vi "xunxian.vi"   [LabVIEW 2015]
uses:
  <vilib>/myRIO/Instrument Drivers/Onboard IO/DIO/typedefs/DIO Reference.ctl
  <vilib>/myRIO/Common/Instrument Driver Framework/Utilities/typedefs/myRIO Generic Hardware Reference.ctl
  <vilib>/myRIO/Common/Instrument Driver Framework/Utilities/typedefs/Hardware Version Enum.ctl
  <vilib>/myRIO/Common/Instrument Driver Framework/Utilities/typedefs/myRIO v1.0 Reference.ctl
  <vilib>/myRIO/Common/Instrument Driver Framework/Utilities/typedefs/Generic FPGA Reference.ctl
  <vilib>/myRIO/Common/Instrument Driver Framework/myRIO v1.0/DIO/typedefs/DIO Channels List.ctl
  <vilib>/myRIO/Common/Instrument Driver Framework/myRIO v1.0/DIO/typedefs/DIO Channels Enum.ctl
  <vilib>/userdefined/High Color/nirio_resource_hc.ctl
  <vilib>/myRIO/Instrument Drivers/Onboard IO/PWM/typedefs/PWM Reference.ctl
  <vilib>/myRIO/Common/Instrument Driver Framework/myRIO v1.0/PWM/typedefs/PWM Channels Enum.ctl
  <vilib>/myRIO/Instrument Drivers/Onboard IO/PWM/typedefs/PWM Configuration.ctl
  <vilib>/myRIO/Common/Instrument Driver Framework/Utilities/vis/Is FPGA Ref Available.vi
  <vilib>/myRIO/Common/Instrument Driver Framework/myRIO v1.0/DIO/vis/myRIO v1.1 Open DIO.vi
  <vilib>/myRIO/Instrument Drivers/Onboard IO/DIO/vis/Read.vi
  <vilib>/myRIO/Instrument Drivers/Onboard IO/DIO/vis/Write.vi
  <vilib>/myRIO/Common/Instrument Driver Framework/myRIO v1.0/PWM/vis/myRIO v1.1 Open PWM.vi
  <vilib>/myRIO/Instrument Drivers/Onboard IO/PWM/vis/Set Duty Cycle and Frequency.vi
  <vilib>/myRIO/Common/Instrument Driver Framework/Utilities/vis/Validate Channels.vi
  <vilib>/myRIO/Common/Instrument Driver Framework/myRIO v1.0/DIO/vis/myRIO v1.0 Reserve DIO.vi
  <vilib>/myRIO/Common/Instrument Driver Framework/myRIO v1.0/PWM/vis/myRIO v1.0 Reserve PWM.vi
  <vilib>/myRIO/Common/Instrument Driver Framework/myRIO v1.0/Resource Manager/vis/myRIO v1.0 Reserve Channel List.vi
  <vilib>/myRIO/Common/Instrument Driver Framework/myRIO v1.0/DIO/vis/myRIO v1.0 Build MUX Configuration DIO.vi
  <vilib>/myRIO/Common/Instrument Driver Framework/myRIO v1.0/PWM/vis/myRIO v1.0 Build MUX Configuration PWM.vi
  <vilib>/myRIO/Common/Instrument Driver Framework/myRIO v1.0/Resource Manager/vis/myRIO v1.0 Reserve Channel.vi
  <vilib>/myRIO/Common/Instrument Driver Framework/myRIO v1.0/Resource Manager/vis/myRIO v1.0 Unreserve Channel.vi
  <vilib>/myRIO/Common/Instrument Driver Framework/myRIO v1.0/Resource Manager/vis/myRIO v1.0 Create Configuration List.vi
  <vilib>/myRIO/Common/Instrument Driver Framework/myRIO v1.0/Resource Manager/vis/myRIO v1.0 Build Mutex Name.vi
  <vilib>/Utility/VariantDataType/GetNumericInfo.vi
  <vilib>/Utility/error.llb/Error Cluster From Error Code.vi
  <vilib>/myRIO/Common/Instrument Driver Framework/myRIO v1.0/myRIO v1.1 Open.vi
  <vilib>/myRIO/Common/Instrument Driver Framework/Utilities/vis/IO Manager.vi
  <vilib>/myRIO/Common/Instrument Driver Framework/Utilities/vis/Configuration Manager.vi
  <vilib>/myRIO/Common/Instrument Driver Framework/myRIO v1.0/Resource Manager/vis/myRIO v1.0 Configure IO.vi
  <vilib>/myRIO/Common/Instrument Driver Framework/myRIO v1.0/myRIO v1.0 Close.vi
  <vilib>/myRIO/Common/Instrument Driver Framework/myRIO v1.0/DIO/vis/myRIO v1.0 Write DIO.vi
  <vilib>/myRIO/Common/Instrument Driver Framework/myRIO v1.0/DIO/vis/myRIO v1.0 Read DIO.vi
  <vilib>/myRIO/Common/Instrument Driver Framework/myRIO v1.0/PWM/vis/myRIO v1.0 Write PWM.vi
  <vilib>/myRIO/Express VI/Onboard IO/DO/DO Express VI.xnode
  <vilib>/myRIO/Instrument Drivers/Onboard IO/DIO/vis/myRIO DIO Open.xnode
  <vilib>/myRIO/Express VI/Onboard IO/DI/DI Express VI.xnode
  <vilib>/myRIO/Express VI/Onboard IO/PWM/PWM Express VI.xnode
  <vilib>/myRIO/Instrument Drivers/Onboard IO/PWM/vis/myRIO PWM Open.xnode
  <vilib>/myRIO/Instrument Drivers/Onboard IO/PWM/PWM.lvlib
  <vilib>/myRIO/Instrument Drivers/Onboard IO/DIO/DIO.lvlib
types:
  T1 = typedef "DIO.lvlib/DIO Reference.ctl" = cluster{"myRIO Reference":T2, "DIO Channels List":T6}
  T2 = typedef "myRIO Generic Hardware Reference.ctl" = cluster{"myRIO Model":T3, "myRIO Hardware Reference":T4}
  T3 = typedef "Hardware Version Enum.ctl" = enum16{"Unknown", "myRIO-1900", "myRIO-1950", "roboRIO"}
  T4 = typedef "myRIO v1.0 Reference.ctl" = cluster{"Generic FPGA Reference":T5, "Allow multiple opens":bool}
  T5 = typedef "Generic FPGA Reference.ctl" = refnum<k20>
  T6 = typedef "DIO Channels List.ctl" = T7[]
  T7 = typedef "DIO Channels Enum.ctl" = enum16{"Not Connected", "C/DIO0", "C/DIO1", "C/DIO2", "C/DIO3", "C/DIO4", "C/DIO5", "C/DIO6", "C/DIO7", "A/DIO0", "A/DIO1", "A/DIO2", "A/DIO3", "A/DIO4", "A/DIO5", "A/DIO6", "A/DIO7", "A/DIO8", "A/DIO9", "A/DIO10", "A/DIO11", "A/DIO12", "A/DIO13", "A/DIO14", "A/DIO15", "B/DIO0", "B/DIO1", "B/DIO2", "B/DIO3", "B/DIO4", "B/DIO5", "B/DIO6", "B/DIO7", "B/DIO8", "B/DIO9", "B/DIO10", "B/DIO11", "B/DIO12", "B/DIO13", "B/DIO14", "B/DIO15", "LED0", "LED1", "LED2", "LED3", "Button0", "DIO/DIO0", "DIO/DIO1", "DIO/DIO2", "DIO/DIO3", "DIO/DIO4", "DIO/DIO5", "DIO/DIO6", "DIO/DIO7", "DIO/DIO8", "DIO/DIO9", "SPI/CS0", "SPI/CS1", "SPI/CS2", "SPI/CS3", "LED RADIO (Green)", "LED RADIO (Red)", "LED COMM (Green)", "LED COMM (Red)", "LED MODE (Green)", "LED MODE (Red)"}
  T8 = typedef "nirio_resource_hc.ctl" = tag
  T9 = typedef "PWM.lvlib/PWM Reference.ctl" = cluster{"myRIO Reference":T2, "PWM Channels Enum":T10, "PWM Configuration":T11}
  T10 = typedef "PWM Channels Enum.ctl" = enum16{"Not Connected", "C/PWM0", "C/PWM1", "A/PWM0", "A/PWM1", "A/PWM2", "B/PWM0", "B/PWM1", "B/PWM2", "PWM/PWM0", "PWM/PWM1", "PWM/PWM2", "PWM/PWM3", "PWM/PWM4", "PWM/PWM5", "PWM/PWM6", "PWM/PWM7", "PWM/PWM8", "PWM/PWM9"}
  T11 = typedef "PWM.lvlib/PWM Configuration.ctl" = cluster{"Frequency":dbl, "Duty Cycle":dbl}
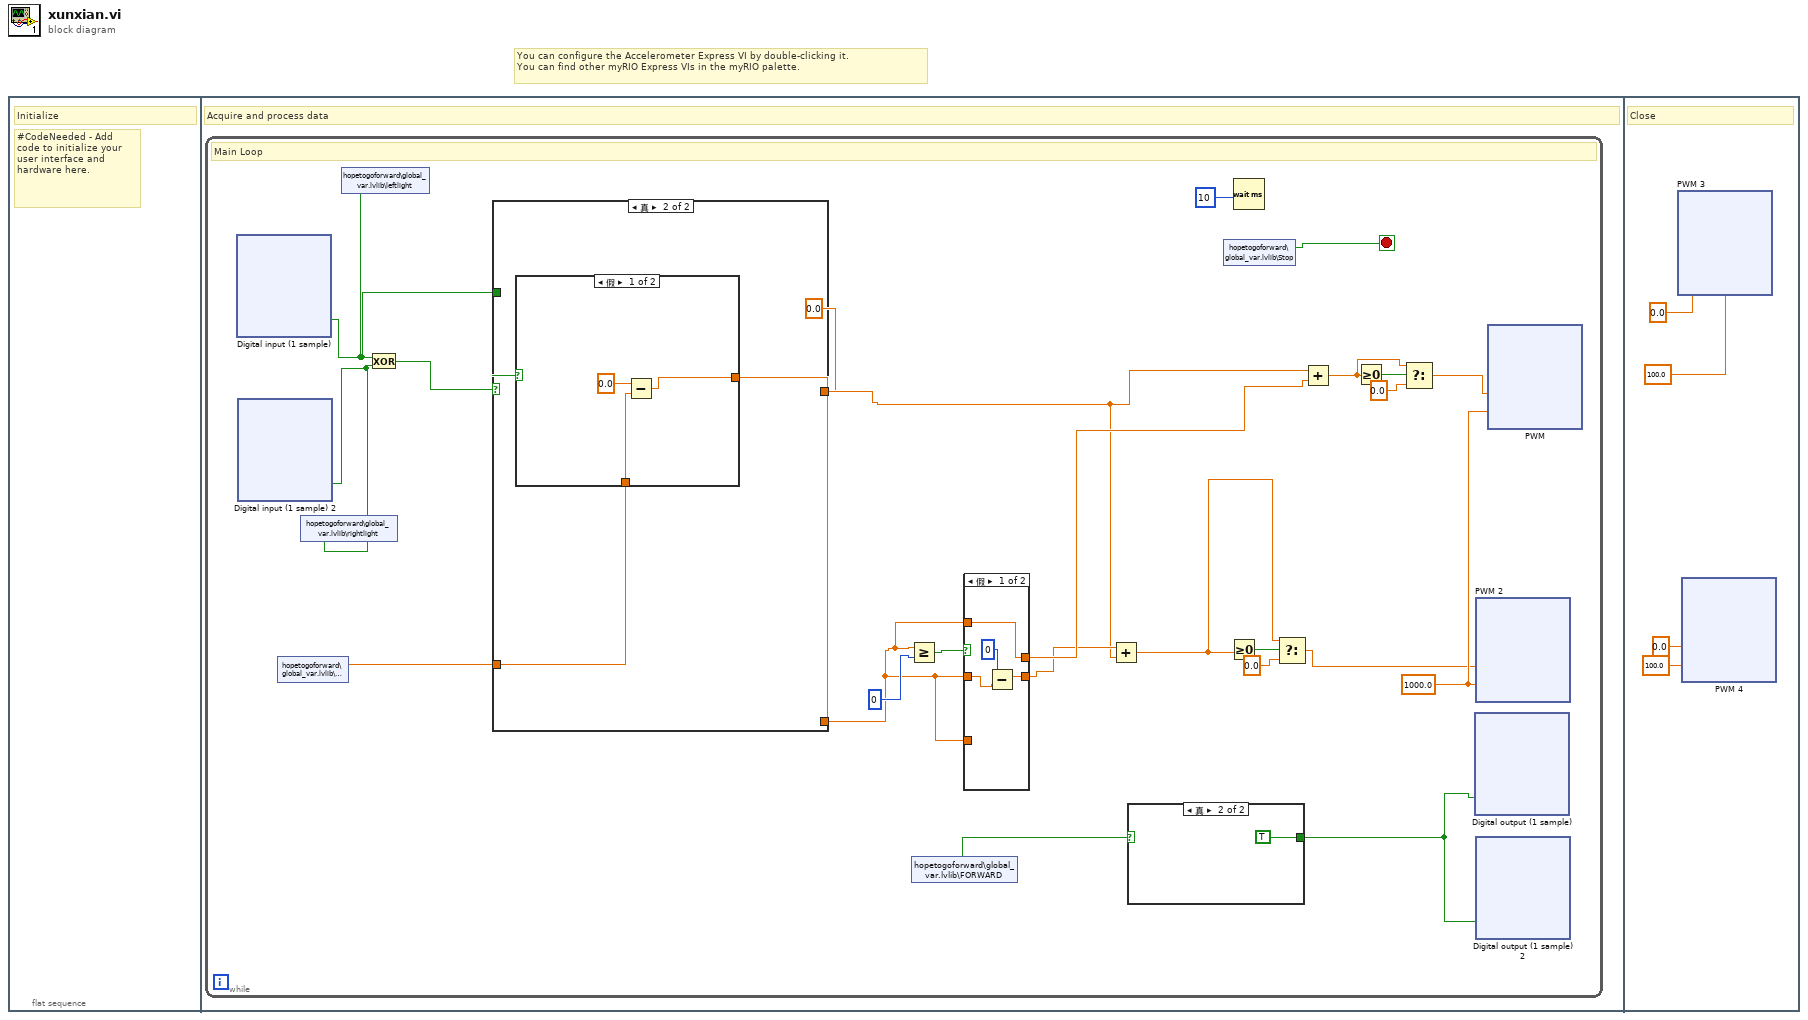
[diagram p0: block diagram]
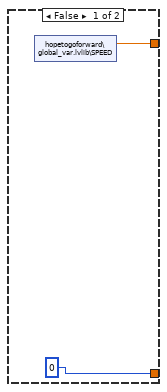
[diagram p2: hidden frame]
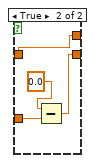
[diagram p4: hidden frame]
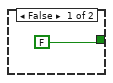
[diagram p5: hidden frame]
diagram:
  # "You can configure the Accelerometer Express VI by double-clicking it.\nYou can find other myRIO Express VIs in the myRIO palette."
  n1 = flat-sequence {
    frame #0 {
      # "#CodeNeeded - Add code to initialize your user interface and hardware here."
      # "Initialize"
    }
    frame #1 {
      # "Acquire and process data"
      n2 = while {
        stop <- w23 stop-if-true
        w21 = 1000.0 ("Frequency [Hz]")
        # "Main Loop"
        n3 = xnode "Digital input (1 sample)"() -> ("C/DIO0 (DIO0)"=w4:bool)  [unwired: 1 in, 1 out]
        n4 = xnode "Digital input (1 sample) 2"() -> ("C/DIO1 (DIO1)"=w3:bool)  [unwired: 1 in, 1 out]
        n5 = shared-variable "hopetogoforward\\global_var.lvlib\\LEFT"() -> (w2:dbl)  [unwired: 1 in, 1 out]
        n6 = shared-variable "hopetogoforward\\global_var.lvlib\\rightlight"(w3) -> ()  [unwired: 1 in, 1 out]
        n7 = shared-variable "hopetogoforward\\global_var.lvlib\\leftlight"(w4) -> ()  [unwired: 1 in, 1 out]
        n8 = Exclusive Or(1:w3, 2:w4) -> (0:w6:bool)
        n9 = case shown="真" w6 {
          tunnel: [0 w28] -> w5
          tunnel: w4 -> [_ w29]
          tunnel: w2 -> [_ w27]
          tunnel: [w24 0.0] -> w1
          frame False {
            n10 = shared-variable "hopetogoforward\\global_var.lvlib\\SPEED"() -> (w24:dbl)  [unwired: 1 in, 1 out]
          }
          frame True {
            n11 = case shown="假" w29 {
              tunnel: [w30 w33] -> w28
              tunnel: w27 -> [w31 w33]
              frame False {
                n12 = Subtract(x=0.0, y=w31) -> (x-y=w30:dbl)
              }
              frame True {
              }
            }
          }
        }
        n13 = Greater Or Equal?(x=w5, y=0) -> (x >= y?=w11:bool)
        n14 = shared-variable "hopetogoforward\\global_var.lvlib\\FORWARD"() -> (w20:bool)  [unwired: 1 in, 1 out]
        n15 = case shown="假" w11 {
          tunnel: w5 -> [w107 w111]
          tunnel: [w104 w111] -> w8
          tunnel: [w105 w108] -> w7
          tunnel: w5 -> [_ w109]
          tunnel: w5 -> [w104 _]
          frame False {
            n16 = Subtract(x=0, y=w107) -> (x-y=w105:dbl)
          }
          frame True {
            n17 = Subtract(x=0.0, y=w109) -> (x-y=w108:dbl)
          }
        }
        n18 = Add(x=w7, y=w1) -> (x+y=w12:dbl)
        n19 = case shown="真" w20 {
          tunnel: [FALSE TRUE] -> w19
          frame False {
          }
          frame True {
          }
        }
        n20 = shared-variable "hopetogoforward\\global_var.lvlib\\Stop"() -> (w23:bool)  [unwired: 1 in, 1 out]
        n21 = Greater Or Equal To 0?(x=w12) -> (x >= 0?=w14:bool)
        n22 = Wait (ms)(milliseconds to wait=u32 10) -> ()  [unwired: 1 out]
        n23 = Select(t=w12, s=w14, f=0.0) -> (s? t:f=w13:dbl)
        n24 = Add(x=w1, y=w8) -> (x+y=w9:dbl)
        n25 = Greater Or Equal To 0?(x=w9) -> (x >= 0?=w18:bool)
        n26 = Select(t=w9, s=w18, f=0.0) -> (s? t:f=w16:dbl)
        n27 = xnode "Digital output (1 sample)"("A/DIO0 (Pin 11)"=w19) -> ()  [unwired: 1 in, 1 out]
        n28 = xnode "PWM 2"("Duty Cycle"=w13, "Frequency [Hz]"=w21) -> ()  [unwired: 1 in, 1 out]
        n29 = xnode "Digital output (1 sample) 2"("A/DIO1 (Pin 13)"=w19) -> ()  [unwired: 1 in, 1 out]
        n30 = xnode "PWM"("Duty Cycle"=w16, "Frequency [Hz]"=w21) -> ()  [unwired: 1 in, 1 out]
      }
    }
    frame #2 {
      # "Close"
      n31 = xnode "PWM 3"("Duty Cycle"=0.0, "Frequency [Hz]"=100.0) -> ()  [unwired: 1 in, 1 out]
      n32 = xnode "PWM 4"("Duty Cycle"=0.0, "Frequency [Hz]"=100.0) -> ()  [unwired: 1 in, 1 out]
    }
  }
